vi "add values.vi"(5 "index string":string, 7 "is array element?":bool, 8 "error in (no error)":errorcluster, 9 "Item Indent":i32, 10 "Variant":variant, 11 "Items in":T1(array[cluster])) -> (0 "error out":errorcluster, 3 "Items out":T1(array[cluster]))   [LabVIEW 2017, in "DSF Configuration Utility.lvlib"]
uses:
  DSF Configuration Utility.lvlib
  get unit string.vi
  <vilib>/Utility/Data Type/Get Numeric Information.vi
  <vilib>/Utility/Data Type/Get Cluster Information.vi
  <vilib>/Utility/LVClass/Get LV Class Name.vi
  <vilib>/Utility/Data Type/Get Fixed-Point Information.vi
  <vilib>/Utility/Data Type/Get Refnum Information.vi
  <vilib>/Utility/Data Type/NI_Data Type.lvlib
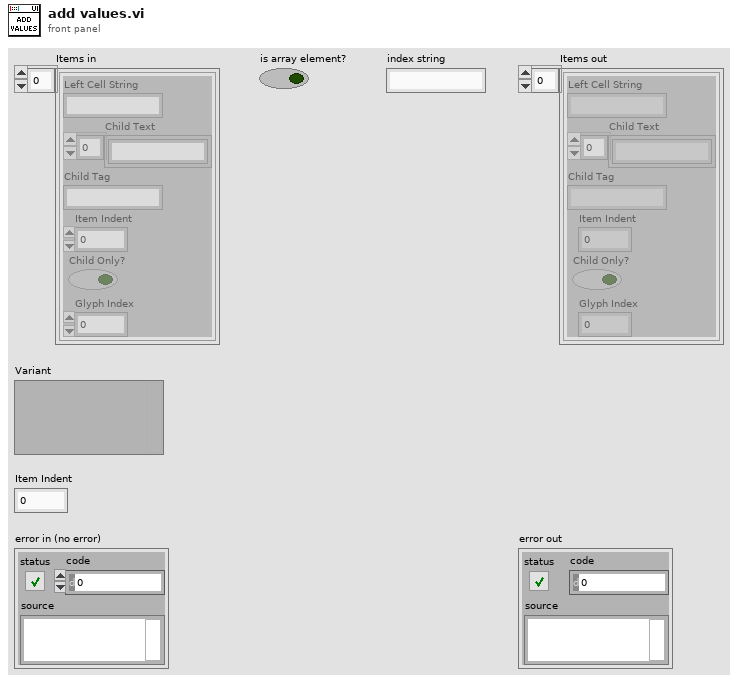
[diagram p1: front panel]
types:
  T1 = cluster{"Left Cell String":string, "Child Text":string[], "Child Tag":string, "Item Indent":i32, "Child Only?":bool, "Glyph Index":i32}[]
  T2 = typedef "NI_Data Type.lvlib/Data Type.ctl" = enum8{"Invalid Type", "Void", "I8", "I16", "I32", "I64", "U8", "U16", "U32", "U64", "Single Float", "Double Float", "Extended Float", "Single Complex", "Double Complex", "Extended Complex", "Enum U8", "Enum U16", "Enum U32", "Enum U64", "Single Float With Unit", "Double Float With Unit", "Extended Float With Unit", "Single Complex with Unit", "Double Complex with Unit", "Extended Complex with Unit", "Boolean", "String", "Path", "Picture", "Tag", "Array", "Cluster", "Variant", "LV Variant", "Waveform", "Timestamp", "Digital Waveform", "Digital Data", "ExpressData", "Refnum", "External Data", "VI", "Poly VI", "LabVIEW Class Instance", "Fixed Point"}
  T3 = cluster{"Left Cell String":string, "Child Text":string[], "Child Tag":string, "Item Indent":i32, "Child Only?":bool, "Glyph Index":i32}
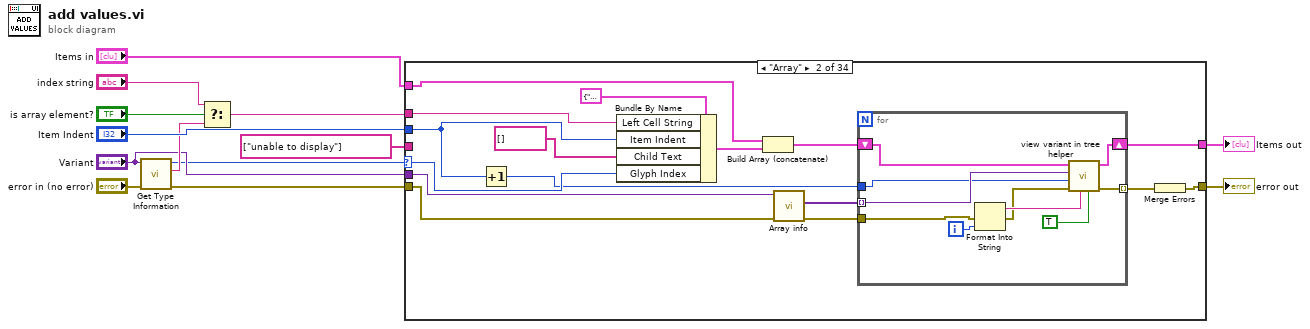
[diagram p0: block diagram]
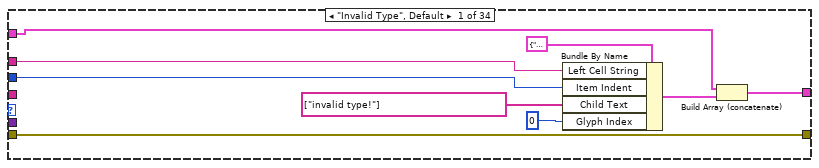
[diagram p2: hidden frame]
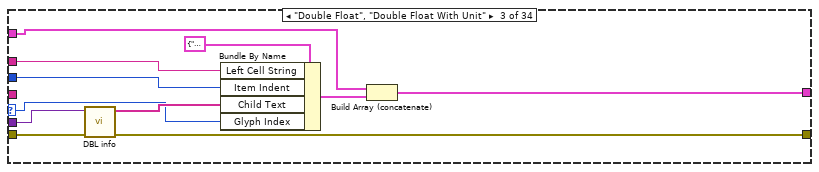
[diagram p3: hidden frame]
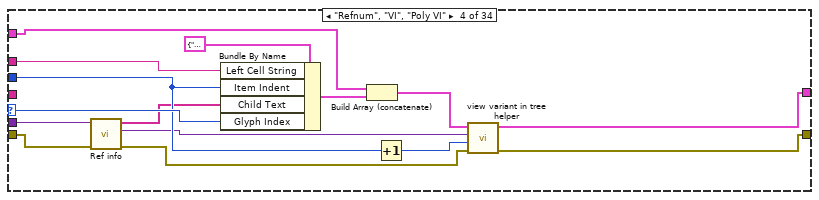
[diagram p4: hidden frame]
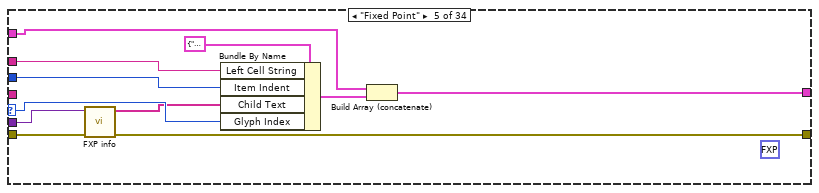
[diagram p5: hidden frame]
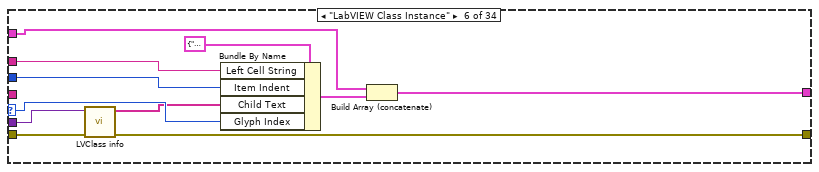
[diagram p6: hidden frame]
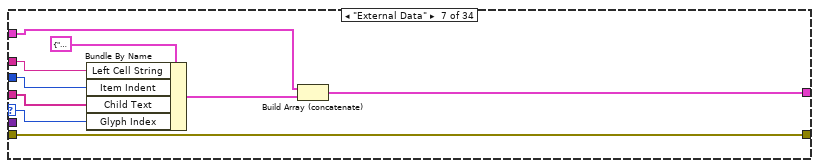
[diagram p7: hidden frame]
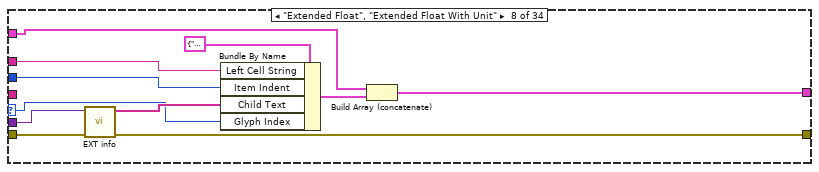
[diagram p8: hidden frame]
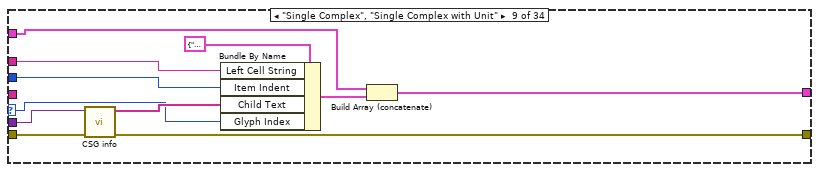
[diagram p9: hidden frame]
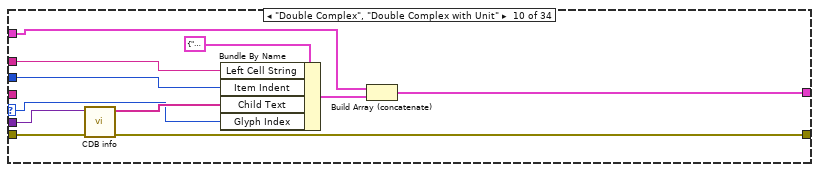
[diagram p10: hidden frame]
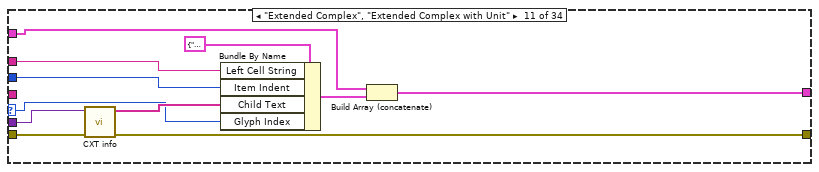
[diagram p11: hidden frame]
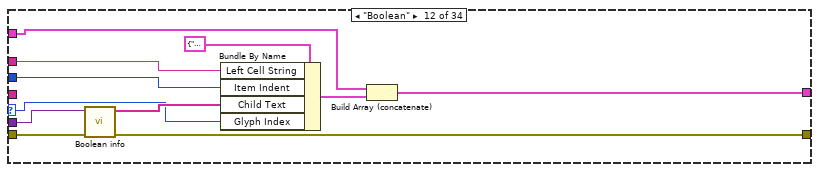
[diagram p12: hidden frame]
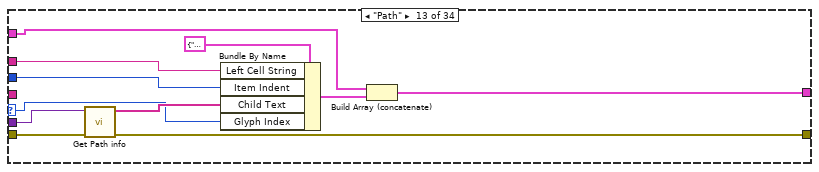
[diagram p13: hidden frame]
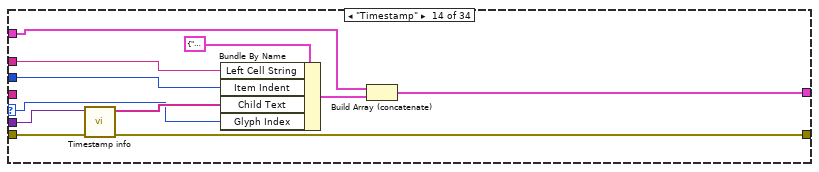
[diagram p14: hidden frame]
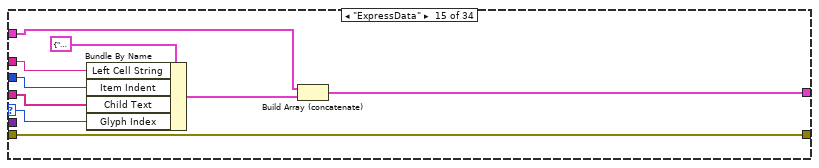
[diagram p15: hidden frame]
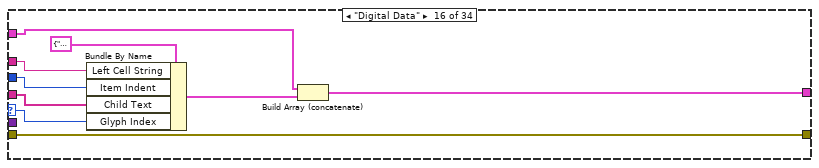
[diagram p16: hidden frame]
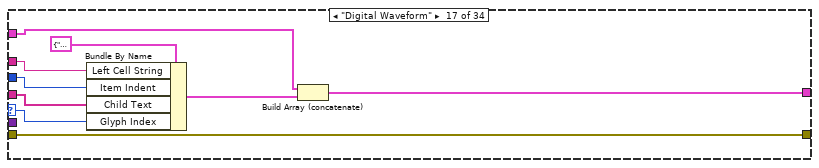
[diagram p17: hidden frame]
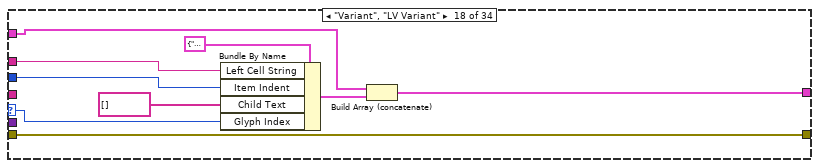
[diagram p18: hidden frame]
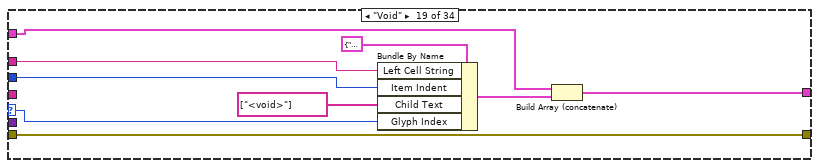
[diagram p19: hidden frame]
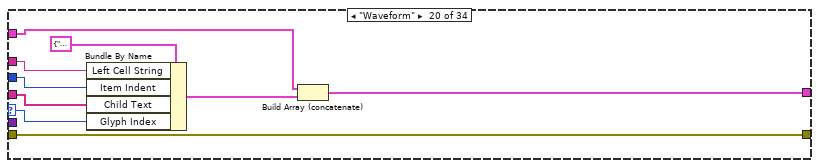
[diagram p20: hidden frame]
diagram:
  n1 = call <vilib>:"Get Type Information.vi"("error in (no error)"="error in (no error)", "Variant"="Variant") -> ("error out"=w12:errorcluster, "Name"=w9:string, "Type"=w4:T2)  [unwired: 5 in, 2 out]
  n2 = Select(t="index string", s="is array element?", f=w9) -> (s? t:f=w1:string)
  n3 = case shown="\"Array\"" w4 {
    selector: w4 -> [_ w29 w53 w71 w79 w90 w99 w109 w120 w131 w142 w152 w163 w174 w184 w193 w202 w212 w221 w229 w243 w260 w269 w279 w290 w302 w312 w323 w334 w345 w356 w367 w378 w389]
    tunnel: "Items in" -> [w17 w35 w56 w69 w82 w93 w102 w112 w123 w134 w145 w155 w166 w177 w188 w197 w206 w216 w225 w233 w250 w264 w273 w282 w295 w306 w317 w328 w339 w350 w361 w372 w383 w394]
    tunnel: "Variant" -> [_ w38 w49 w70 w76 w87 _ w108 w118 w129 w140 w157 w168 w179 _ _ _ _ _ _ w244 _ _ w284 w292 w301 w314 w325 w336 w347 w358 w369 w380 w391]
    tunnel: w1 -> [w14 w30 w50 w73 w84 w95 w104 w115 w126 w137 w148 w159 w170 w181 w190 w199 w208 w217 w226 w235 w251 w266 w275 w286 w297 w308 w319 w330 w341 w352 w363 w374 w385 w396]
    tunnel: "Item Indent" -> [w20 w36 w58 w66 w83 w94 w103 w114 w125 w136 w147 w158 w169 w180 w189 w198 w207 w213 w222 w234 w246 w265 w274 w285 w296 w307 w318 w329 w340 w351 w362 w373 w384 w395]
    tunnel: [w15 w32 w54 w67 w80 w91 w100 w110 w121 w132 w143 w153 w164 w175 w186 w195 w204 w214 w223 w231 w247 w262 w271 w280 w293 w304 w315 w326 w337 w348 w359 w370 w381 w392] -> w8
    tunnel: string[] ["unable to display"] ("Child Text") -> [_ _ _ _ _ _ w97 _ _ _ _ _ _ _ w185 w194 w203 _ _ w230 _ w261 w270 _ _ _ _ _ _ _ _ _ _ _]
    tunnel: w12 -> [w22 w28 w52 w61 w78 w89 w98 w107 w119 w128 w141 w151 w162 w173 w183 w192 w201 w211 w220 w228 w242 w259 w268 w278 w289 w300 w311 w322 w333 w344 w355 w366 w377 w388]
    tunnel: [w22 w25 w51 w64 w77 w88 w98 w106 w117 w130 w139 w150 w161 w172 w183 w192 w201 w211 w220 w228 w239 w259 w268 w277 w288 w299 w310 w321 w332 w343 w354 w365 w376 w387] -> w13
    frame "Invalid Type", Default {
      n4 = Bundle By Name(cluster=T3 {"Left Cell String"="", "Child Text"=[], "Child Tag"="", "Item Indent"=0, "Child Only?"=FALSE, "Glyph Index"=0} ("Item"), "Left Cell String"=w14, "Item Indent"=w20, "Child Text"=string[] ["invalid type!"], "Glyph Index"=0) -> (w16:T3)
      n5 = Build Array (concatenate)(w17, w16) -> (w15:T1)
    }
    frame "Array" {
      n6 = Increment(x=w36) -> (x+1=w23:i32)
      n7 = Bundle By Name(cluster=T3 {"Left Cell String"="", "Child Text"=[], "Child Tag"="", "Item Indent"=0, "Child Only?"=FALSE, "Glyph Index"=0} ("Item"), "Left Cell String"=w30, "Item Indent"=w36, "Child Text"=string[] [], "Glyph Index"=w29) -> (w34:T3)
      n8 = Build Array (concatenate)(w35, w34) -> (w33:T1)
      n9 = call "Array info.vi"("error in (no error)"=w28, "Variant"=w38) -> ("error out"=w27:errorcluster, "elements"=w31:variant[])  [unwired: 7 in, 1 out]
      n10 = for {
        tunnel: w31 -> [w46] mode=indexing
        shift-right: [w47] -> w32
        shift-left: w33 -> [w48]
        tunnel: w23 -> [w45]
        tunnel: w27 -> [w41]
        tunnel: [w39] -> w26 mode=indexing
        i -> [w44]
        n11 = Format Into String(error in=w41, w44) -> (resulting string=w43:string, error out=w40:errorcluster)  [unwired: 2 in]
        n12 = call "view variant in tree helper.vi"("is array element?"=TRUE, "index string"=w43, "error in (no error)"=w40, "Item Indent"=w45, "Variant"=w46, "Items"=w48) -> ("error out"=w39:errorcluster, "Items out"=w47:T1)  [unwired: 4 in]
      }
      n13 = Merge Errors(w26) -> (w25:errorcluster)
    }
    frame "Double Float", "Double Float With Unit" {
      n14 = call "DBL info.vi"("error in (no error)"=w52, "Variant"=w49) -> ("error out"=w51:errorcluster, "child strings"=w57:string[])  [unwired: 8 in]
      n15 = Bundle By Name(cluster=T3 {"Left Cell String"="", "Child Text"=[], "Child Tag"="", "Item Indent"=0, "Child Only?"=FALSE, "Glyph Index"=0} ("Item"), "Left Cell String"=w50, "Item Indent"=w58, "Child Text"=w57, "Glyph Index"=w53) -> (w55:T3)
      n16 = Build Array (concatenate)(w56, w55) -> (w54:T1)
    }
    frame "Refnum", "VI", "Poly VI" {
      n17 = call "Ref info.vi"("error in (no error)"=w61, "Variant"=w70) -> ("error out"=w60:errorcluster, "refnum type"=w62:variant, "child strings"=w63:string[])  [unwired: 7 in]
      n18 = Bundle By Name(cluster=T3 {"Left Cell String"="", "Child Text"=[], "Child Tag"="", "Item Indent"=0, "Child Only?"=FALSE, "Glyph Index"=0} ("Item"), "Left Cell String"=w73, "Item Indent"=w66, "Child Text"=w63, "Glyph Index"=w71) -> (w72:T3)
      n19 = Build Array (concatenate)(w69, w72) -> (w68:T1)
      n20 = Increment(x=w66) -> (x+1=w65:i32)
      n21 = call "view variant in tree helper.vi"("error in (no error)"=w60, "Item Indent"=w65, "Variant"=w62, "Items"=w68) -> ("error out"=w64:errorcluster, "Items out"=w67:T1)  [unwired: 6 in]
    }
    frame "Fixed Point" {
      (unwired) fxp<+,1,1> 0.0
      n22 = call "FXP info.vi"("error in (no error)"=w78, "Variant"=w76) -> ("error out"=w77:errorcluster, "child strings"=w75:string[])  [unwired: 8 in]
      n23 = Bundle By Name(cluster=T3 {"Left Cell String"="", "Child Text"=[], "Child Tag"="", "Item Indent"=0, "Child Only?"=FALSE, "Glyph Index"=0} ("Item"), "Left Cell String"=w84, "Item Indent"=w83, "Child Text"=w75, "Glyph Index"=w79) -> (w81:T3)
      n24 = Build Array (concatenate)(w82, w81) -> (w80:T1)
    }
    frame "LabVIEW Class Instance" {
      n25 = call "LVClass info.vi"("error in (no error)"=w89, "Variant"=w87) -> ("error out"=w88:errorcluster, "child strings"=w86:string[])  [unwired: 8 in]
      n26 = Bundle By Name(cluster=T3 {"Left Cell String"="", "Child Text"=[], "Child Tag"="", "Item Indent"=0, "Child Only?"=FALSE, "Glyph Index"=0} ("Item"), "Left Cell String"=w95, "Item Indent"=w94, "Child Text"=w86, "Glyph Index"=w90) -> (w92:T3)
      n27 = Build Array (concatenate)(w93, w92) -> (w91:T1)
    }
    frame "External Data" {
      n28 = Bundle By Name(cluster=T3 {"Left Cell String"="", "Child Text"=[], "Child Tag"="", "Item Indent"=0, "Child Only?"=FALSE, "Glyph Index"=0} ("Item"), "Left Cell String"=w104, "Item Indent"=w103, "Child Text"=w97, "Glyph Index"=w99) -> (w101:T3)
      n29 = Build Array (concatenate)(w102, w101) -> (w100:T1)
    }
    frame "Extended Float", "Extended Float With Unit" {
      n30 = call "EXT info.vi"("error in (no error)"=w107, "Variant"=w108) -> ("error out"=w106:errorcluster, "child strings"=w113:string[])  [unwired: 8 in]
      n31 = Bundle By Name(cluster=T3 {"Left Cell String"="", "Child Text"=[], "Child Tag"="", "Item Indent"=0, "Child Only?"=FALSE, "Glyph Index"=0} ("Item"), "Left Cell String"=w115, "Item Indent"=w114, "Child Text"=w113, "Glyph Index"=w109) -> (w111:T3)
      n32 = Build Array (concatenate)(w112, w111) -> (w110:T1)
    }
    frame "Single Complex", "Single Complex with Unit" {
      n33 = call "CSG info.vi"("error in (no error)"=w119, "Variant"=w118) -> ("error out"=w117:errorcluster, "child strings"=w124:string[])  [unwired: 8 in]
      n34 = Bundle By Name(cluster=T3 {"Left Cell String"="", "Child Text"=[], "Child Tag"="", "Item Indent"=0, "Child Only?"=FALSE, "Glyph Index"=0} ("Item"), "Left Cell String"=w126, "Item Indent"=w125, "Child Text"=w124, "Glyph Index"=w120) -> (w122:T3)
      n35 = Build Array (concatenate)(w123, w122) -> (w121:T1)
    }
    frame "Double Complex", "Double Complex with Unit" {
      n36 = call "CDB info.vi"("error in (no error)"=w128, "Variant"=w129) -> ("error out"=w130:errorcluster, "child strings"=w135:string[])  [unwired: 8 in]
      n37 = Bundle By Name(cluster=T3 {"Left Cell String"="", "Child Text"=[], "Child Tag"="", "Item Indent"=0, "Child Only?"=FALSE, "Glyph Index"=0} ("Item"), "Left Cell String"=w137, "Item Indent"=w136, "Child Text"=w135, "Glyph Index"=w131) -> (w133:T3)
      n38 = Build Array (concatenate)(w134, w133) -> (w132:T1)
    }
    frame "Extended Complex", "Extended Complex with Unit" {
      n39 = call "CXT info.vi"("error in (no error)"=w141, "Variant"=w140) -> ("error out"=w139:errorcluster, "child strings"=w146:string[])  [unwired: 8 in]
      n40 = Bundle By Name(cluster=T3 {"Left Cell String"="", "Child Text"=[], "Child Tag"="", "Item Indent"=0, "Child Only?"=FALSE, "Glyph Index"=0} ("Item"), "Left Cell String"=w148, "Item Indent"=w147, "Child Text"=w146, "Glyph Index"=w142) -> (w144:T3)
      n41 = Build Array (concatenate)(w145, w144) -> (w143:T1)
    }
    frame "Boolean" {
      n42 = call "Boolean info.vi"("error in (no error)"=w151, "Variant"=w157) -> ("error out"=w150:errorcluster, "child strings"=w156:string[])  [unwired: 8 in]
      n43 = Bundle By Name(cluster=T3 {"Left Cell String"="", "Child Text"=[], "Child Tag"="", "Item Indent"=0, "Child Only?"=FALSE, "Glyph Index"=0} ("Item"), "Left Cell String"=w159, "Item Indent"=w158, "Child Text"=w156, "Glyph Index"=w152) -> (w154:T3)
      n44 = Build Array (concatenate)(w155, w154) -> (w153:T1)
    }
    frame "Path" {
      n45 = call "Get Path info.vi"("error in (no error)"=w162, "Variant"=w168) -> ("error out"=w161:errorcluster, "child strings"=w167:string[])  [unwired: 8 in]
      n46 = Bundle By Name(cluster=T3 {"Left Cell String"="", "Child Text"=[], "Child Tag"="", "Item Indent"=0, "Child Only?"=FALSE, "Glyph Index"=0} ("Item"), "Left Cell String"=w170, "Item Indent"=w169, "Child Text"=w167, "Glyph Index"=w163) -> (w165:T3)
      n47 = Build Array (concatenate)(w166, w165) -> (w164:T1)
    }
    frame "Timestamp" {
      n48 = call "Timestamp info.vi"("error in (no error)"=w173, "Variant"=w179) -> ("error out"=w172:errorcluster, "child strings"=w178:string[])  [unwired: 8 in]
      n49 = Bundle By Name(cluster=T3 {"Left Cell String"="", "Child Text"=[], "Child Tag"="", "Item Indent"=0, "Child Only?"=FALSE, "Glyph Index"=0} ("Item"), "Left Cell String"=w181, "Item Indent"=w180, "Child Text"=w178, "Glyph Index"=w174) -> (w176:T3)
      n50 = Build Array (concatenate)(w177, w176) -> (w175:T1)
    }
    frame "ExpressData" {
      n51 = Bundle By Name(cluster=T3 {"Left Cell String"="", "Child Text"=[], "Child Tag"="", "Item Indent"=0, "Child Only?"=FALSE, "Glyph Index"=0} ("Item"), "Left Cell String"=w190, "Item Indent"=w189, "Child Text"=w185, "Glyph Index"=w184) -> (w187:T3)
      n52 = Build Array (concatenate)(w188, w187) -> (w186:T1)
    }
    frame "Digital Data" {
      n53 = Bundle By Name(cluster=T3 {"Left Cell String"="", "Child Text"=[], "Child Tag"="", "Item Indent"=0, "Child Only?"=FALSE, "Glyph Index"=0} ("Item"), "Left Cell String"=w199, "Item Indent"=w198, "Child Text"=w194, "Glyph Index"=w193) -> (w196:T3)
      n54 = Build Array (concatenate)(w197, w196) -> (w195:T1)
    }
    frame "Digital Waveform" {
      n55 = Bundle By Name(cluster=T3 {"Left Cell String"="", "Child Text"=[], "Child Tag"="", "Item Indent"=0, "Child Only?"=FALSE, "Glyph Index"=0} ("Item"), "Left Cell String"=w208, "Item Indent"=w207, "Child Text"=w203, "Glyph Index"=w202) -> (w205:T3)
      n56 = Build Array (concatenate)(w206, w205) -> (w204:T1)
    }
    frame "Variant", "LV Variant" {
      n57 = Bundle By Name(cluster=T3 {"Left Cell String"="", "Child Text"=[], "Child Tag"="", "Item Indent"=0, "Child Only?"=FALSE, "Glyph Index"=0} ("Item"), "Left Cell String"=w217, "Item Indent"=w213, "Child Text"=string[] [], "Glyph Index"=w212) -> (w215:T3)
      n58 = Build Array (concatenate)(w216, w215) -> (w214:T1)
    }
    frame "Void" {
      n59 = Bundle By Name(cluster=T3 {"Left Cell String"="", "Child Text"=[], "Child Tag"="", "Item Indent"=0, "Child Only?"=FALSE, "Glyph Index"=0} ("Item"), "Left Cell String"=w226, "Item Indent"=w222, "Child Text"=string[] ["<void>"], "Glyph Index"=w221) -> (w224:T3)
      n60 = Build Array (concatenate)(w225, w224) -> (w223:T1)
    }
    frame "Waveform" {
      n61 = Bundle By Name(cluster=T3 {"Left Cell String"="", "Child Text"=[], "Child Tag"="", "Item Indent"=0, "Child Only?"=FALSE, "Glyph Index"=0} ("Item"), "Left Cell String"=w235, "Item Indent"=w234, "Child Text"=w230, "Glyph Index"=w229) -> (w232:T3)
      n62 = Build Array (concatenate)(w233, w232) -> (w231:T1)
    }
    frame "Cluster" {
      n63 = Increment(x=w246) -> (x+1=w237:i32)
      n64 = Bundle By Name(cluster=T3 {"Left Cell String"="", "Child Text"=[], "Child Tag"="", "Item Indent"=0, "Child Only?"=FALSE, "Glyph Index"=0} ("Item"), "Left Cell String"=w251, "Item Indent"=w246, "Child Text"=string[] [], "Glyph Index"=w243) -> (w249:T3)
      n65 = call "Variant Cluster to Array.vi"("error in (no error)"=w242, "Cluster"=w244) -> ("error out"=w241:errorcluster, "Array"=w245:variant[])  [unwired: 8 in]
      n66 = Array Size(array=w245) -> ()  [unwired: 1 out]
      n67 = Build Array (concatenate)(w250, w249) -> (w248:T1)
      n68 = for {
        tunnel: w245 -> [w257] mode=indexing
        shift-right: [w256] -> w247
        shift-left: w248 -> [w258]
        tunnel: w237 -> [w255]
        tunnel: w241 -> [w254]
        tunnel: [w253] -> w240 mode=indexing
        n69 = call "view variant in tree helper.vi"("error in (no error)"=w254, "Item Indent"=w255, "Variant"=w257, "Items"=w258) -> ("error out"=w253:errorcluster, "Items out"=w256:T1)  [unwired: 6 in]
      }
      n70 = Merge Errors(w240) -> (w239:errorcluster)
    }
    frame "Tag" {
      n71 = Bundle By Name(cluster=T3 {"Left Cell String"="", "Child Text"=[], "Child Tag"="", "Item Indent"=0, "Child Only?"=FALSE, "Glyph Index"=0} ("Item"), "Left Cell String"=w266, "Item Indent"=w265, "Child Text"=w261, "Glyph Index"=w260) -> (w263:T3)
      n72 = Build Array (concatenate)(w264, w263) -> (w262:T1)
    }
    frame "Picture" {
      n73 = Bundle By Name(cluster=T3 {"Left Cell String"="", "Child Text"=[], "Child Tag"="", "Item Indent"=0, "Child Only?"=FALSE, "Glyph Index"=0} ("Item"), "Left Cell String"=w275, "Item Indent"=w274, "Child Text"=w270, "Glyph Index"=w269) -> (w272:T3)
      n74 = Build Array (concatenate)(w273, w272) -> (w271:T1)
    }
    frame "String" {
      n75 = call "String info.vi"("error in (no error)"=w278, "Variant"=w284) -> ("error out"=w277:errorcluster, "child strings"=w283:string[])  [unwired: 8 in]
      n76 = Bundle By Name(cluster=T3 {"Left Cell String"="", "Child Text"=[], "Child Tag"="", "Item Indent"=0, "Child Only?"=FALSE, "Glyph Index"=0} ("Item"), "Left Cell String"=w286, "Item Indent"=w285, "Child Text"=w283, "Glyph Index"=w279) -> (w281:T3)
      n77 = Build Array (concatenate)(w282, w281) -> (w280:T1)
    }
    frame "Enum U8".."Enum U64" {
      n78 = call "Enum info.vi"("error in (no error)"=w289, "Variant"=w292) -> ("error out"=w288:errorcluster, "child strings"=w291:string[])  [unwired: 8 in]
      n79 = Bundle By Name(cluster=T3 {"Left Cell String"="", "Child Text"=[], "Child Tag"="", "Item Indent"=0, "Child Only?"=FALSE, "Glyph Index"=0} ("Item"), "Left Cell String"=w297, "Item Indent"=w296, "Child Text"=w291, "Glyph Index"=w290) -> (w294:T3)
      n80 = Build Array (concatenate)(w295, w294) -> (w293:T1)
    }
    frame "Single Float", "Single Float With Unit" {
      n81 = call "SGL info.vi"("error in (no error)"=w300, "Variant"=w301) -> ("error out"=w299:errorcluster, "child strings"=w303:string[])  [unwired: 8 in]
      n82 = Bundle By Name(cluster=T3 {"Left Cell String"="", "Child Text"=[], "Child Tag"="", "Item Indent"=0, "Child Only?"=FALSE, "Glyph Index"=0} ("Item"), "Left Cell String"=w308, "Item Indent"=w307, "Child Text"=w303, "Glyph Index"=w302) -> (w305:T3)
      n83 = Build Array (concatenate)(w306, w305) -> (w304:T1)
    }
    frame "I8" {
      n84 = call "I8 info.vi"("error in (no error)"=w311, "Variant"=w314) -> ("error out"=w310:errorcluster, "child strings"=w313:string[])  [unwired: 8 in]
      n85 = Bundle By Name(cluster=T3 {"Left Cell String"="", "Child Text"=[], "Child Tag"="", "Item Indent"=0, "Child Only?"=FALSE, "Glyph Index"=0} ("Item"), "Left Cell String"=w319, "Item Indent"=w318, "Child Text"=w313, "Glyph Index"=w312) -> (w316:T3)
      n86 = Build Array (concatenate)(w317, w316) -> (w315:T1)
    }
    frame "I16" {
      n87 = call "I16 info.vi"("error in (no error)"=w322, "Variant"=w325) -> ("error out"=w321:errorcluster, "child strings"=w324:string[])  [unwired: 8 in]
      n88 = Bundle By Name(cluster=T3 {"Left Cell String"="", "Child Text"=[], "Child Tag"="", "Item Indent"=0, "Child Only?"=FALSE, "Glyph Index"=0} ("Item"), "Left Cell String"=w330, "Item Indent"=w329, "Child Text"=w324, "Glyph Index"=w323) -> (w327:T3)
      n89 = Build Array (concatenate)(w328, w327) -> (w326:T1)
    }
    frame "I32" {
      n90 = call "I32.vi"("error in (no error)"=w333, "Variant"=w336) -> ("error out"=w332:errorcluster, "child strings"=w335:string[])  [unwired: 8 in]
      n91 = Bundle By Name(cluster=T3 {"Left Cell String"="", "Child Text"=[], "Child Tag"="", "Item Indent"=0, "Child Only?"=FALSE, "Glyph Index"=0} ("Item"), "Left Cell String"=w341, "Item Indent"=w340, "Child Text"=w335, "Glyph Index"=w334) -> (w338:T3)
      n92 = Build Array (concatenate)(w339, w338) -> (w337:T1)
    }
    frame "I64" {
      n93 = call "I64 info.vi"("error in (no error)"=w344, "Variant"=w347) -> ("error out"=w343:errorcluster, "child strings"=w346:string[])  [unwired: 8 in]
      n94 = Bundle By Name(cluster=T3 {"Left Cell String"="", "Child Text"=[], "Child Tag"="", "Item Indent"=0, "Child Only?"=FALSE, "Glyph Index"=0} ("Item"), "Left Cell String"=w352, "Item Indent"=w351, "Child Text"=w346, "Glyph Index"=w345) -> (w349:T3)
      n95 = Build Array (concatenate)(w350, w349) -> (w348:T1)
    }
    frame "U8" {
      n96 = call "U8 info.vi"("error in (no error)"=w355, "Variant"=w358) -> ("error out"=w354:errorcluster, "child strings"=w357:string[])  [unwired: 8 in]
      n97 = Bundle By Name(cluster=T3 {"Left Cell String"="", "Child Text"=[], "Child Tag"="", "Item Indent"=0, "Child Only?"=FALSE, "Glyph Index"=0} ("Item"), "Left Cell String"=w363, "Item Indent"=w362, "Child Text"=w357, "Glyph Index"=w356) -> (w360:T3)
      n98 = Build Array (concatenate)(w361, w360) -> (w359:T1)
    }
    frame "U16" {
      n99 = call "U16 info.vi"("error in (no error)"=w366, "Variant"=w369) -> ("error out"=w365:errorcluster, "child strings"=w368:string[])  [unwired: 8 in]
      n100 = Bundle By Name(cluster=T3 {"Left Cell String"="", "Child Text"=[], "Child Tag"="", "Item Indent"=0, "Child Only?"=FALSE, "Glyph Index"=0} ("Item"), "Left Cell String"=w374, "Item Indent"=w373, "Child Text"=w368, "Glyph Index"=w367) -> (w371:T3)
      n101 = Build Array (concatenate)(w372, w371) -> (w370:T1)
    }
    frame "U32" {
      n102 = call "U32 info.vi"("error in (no error)"=w377, "Variant"=w380) -> ("error out"=w376:errorcluster, "child strings"=w379:string[])  [unwired: 8 in]
      n103 = Bundle By Name(cluster=T3 {"Left Cell String"="", "Child Text"=[], "Child Tag"="", "Item Indent"=0, "Child Only?"=FALSE, "Glyph Index"=0} ("Item"), "Left Cell String"=w385, "Item Indent"=w384, "Child Text"=w379, "Glyph Index"=w378) -> (w382:T3)
      n104 = Build Array (concatenate)(w383, w382) -> (w381:T1)
    }
    frame "U64" {
      n105 = call "U64 info.vi"("error in (no error)"=w388, "Variant"=w391) -> ("error out"=w387:errorcluster, "child strings"=w390:string[])  [unwired: 8 in]
      n106 = Bundle By Name(cluster=T3 {"Left Cell String"="", "Child Text"=[], "Child Tag"="", "Item Indent"=0, "Child Only?"=FALSE, "Glyph Index"=0} ("Item"), "Left Cell String"=w396, "Item Indent"=w395, "Child Text"=w390, "Glyph Index"=w389) -> (w393:T3)
      n107 = Build Array (concatenate)(w394, w393) -> (w392:T1)
    }
  }
  "error out" <- w13
  "Items out" <- w8
